vi "fpga_stop.vi"(8 "error in":errorcluster, 10 "Timeout (ms)":u32=1000, 11 "FPGA VI Reference in":T1) -> (0 "error out":errorcluster, 2 "Timed out?":bool, 3 "FPGA VI Reference out":T1)   [LabVIEW 2011, in "Fiberscope_library.lvlib"]
uses:
  Fiberscope_library.lvlib
  typedefs/fpga_main_spiral_fpga_ref.ctl
  <vilib>/Utility/error.llb/Error Cluster From Error Code.vi
  <vilib>/rvi/errors/niLvFpgaAdjustHostInterfaceError.vi
  <vilib>/rvi/interface/nirviReadWriteControl/nirviReadWriteControl.xnode
  FPGA Bitfiles/FiberscopeRK1107_FPGATarget_fpgamainspiral_0DF2A7CB.lvbitx
  NiFpgaLv.dll
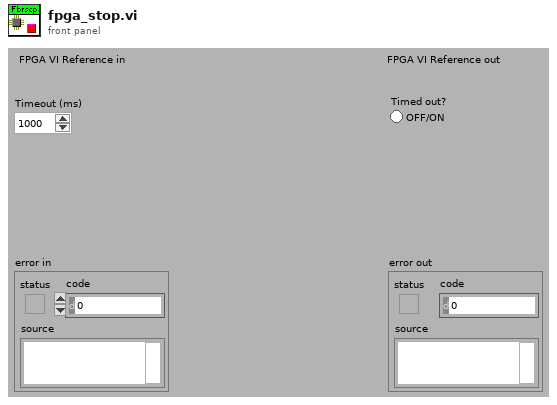
[diagram p1: front panel]
types:
  T1 = typedef "Fiberscope_library.lvlib/fpga_main_spiral_fpga_ref.ctl" = refnum<k20>
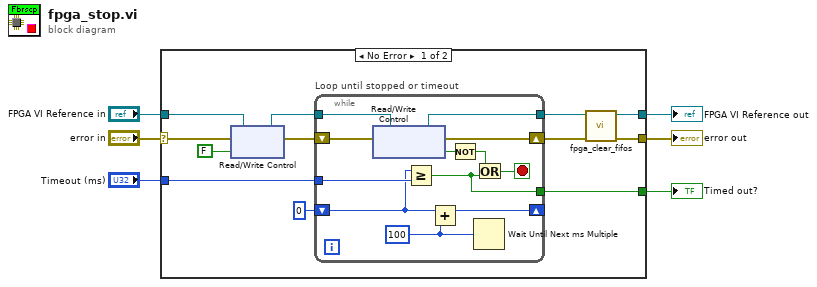
[diagram p0: block diagram]
diagram:
  n1 = case shown="No Error" "error in" {
    selector: "error in" -> [w17 w32]
    tunnel: [w12 w32] -> w5
    tunnel: "FPGA VI Reference in" -> [w18 w31]
    tunnel: [w10 w31] -> w3
    tunnel: "Timeout (ms)" -> [w9 _]
    tunnel: [w7 _] -> w1
    frame No Error {
      n2 = xnode "Read/Write Control"("FPGA VI Reference In"=w18, "error in"=w17, "Scan"=FALSE) -> ("FPGA VI Reference Out"=w14:T1, "error out"=w15:errorcluster)
      n3 = while "Loop until stopped or timeout" {
        shift-right: [w28] -> w13
        shift-left: w15 -> [w30]
        tunnel: w14 -> [w29]
        tunnel: [w24] -> w11
        shift-right: [w23] -> _
        shift-left: u32 0 -> [w21]
        tunnel: w9 -> [w22]
        tunnel: [w19] -> w7
        stop <- w25 stop-if-true
        w20 = u32 100 ("millisecond multiple")
        n4 = xnode "Read/Write Control"("FPGA VI Reference In"=w29, "error in"=w30) -> ("FPGA VI Reference Out"=w24:T1, "error out"=w28:errorcluster, "Scanning?"=w27:bool)
        n5 = Greater Or Equal?(x=w21, y=w22) -> (x >= y?=w19:bool)
        n6 = Add(x=w21, y=w20) -> (x+y=w23:u32)
        n7 = Not(x=w27) -> (.not. x?=w26:bool)
        n8 = Wait Until Next ms Multiple(millisecond multiple=w20) -> ()  [unwired: 1 out]
        n9 = Or(x=w26, y=w19) -> (x .or. y?=w25:bool)
      }
      n10 = call "fpga_clear_fifos.vi"("error in"=w13, "FPGA VI Reference in"=w11) -> ("error out"=w12:errorcluster, "FPGA VI Reference Out"=w10:T1)  [unwired: 8 in]
    }
    frame Error {
    }
  }
  "error out" <- w5
  "FPGA VI Reference out" <- w3
  "Timed out?" <- w1
